vi "Get Antidoc Project Classes.vi"(8 "error in (no error)":errorcluster) -> (0 "error out":errorcluster, 2 "Config":refnum<class "Config.lvclass">, 3 "Document Type out":refnum<class "Document Type.lvclass">)   [LabVIEW 2020, in "CICD.lvlib"]
uses:
  CICD.lvlib
  <vilib>/Wovalab/AntiDoc/Document Type/Document/Document Type.lvclass
  <vilib>/Wovalab/AntiDoc/Document Type/Config/Config.lvclass
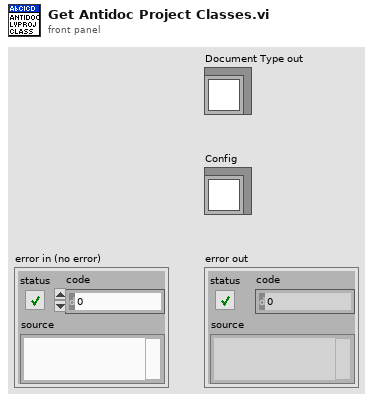
[diagram p1: front panel]
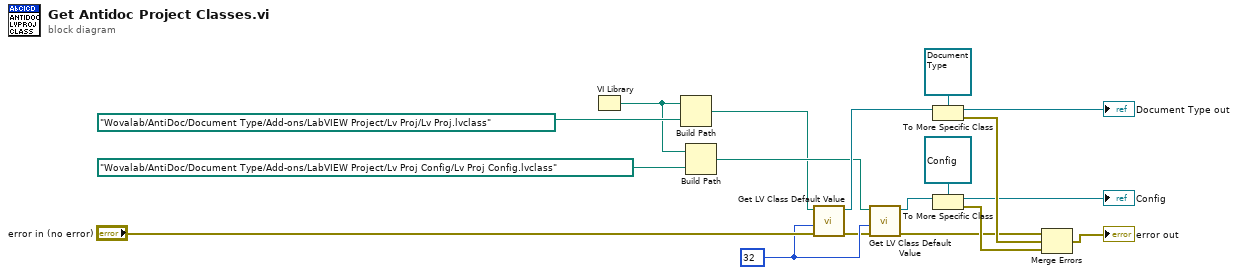
[diagram p0: block diagram]
diagram:
  w5 = u32 32 ("options")
  n1 = VI Library() -> (path=w1:path)
  n2 = Build Path(base path=w1, name or relative path=path "Wovalab/AntiDoc/Document Type/Add-ons/LabVIEW Project/Lv Proj/Lv Proj.lvclass") -> (appended path=w7:path)
  n3 = Build Path(base path=w1, name or relative path=path "Wovalab/AntiDoc/Document Type/Add-ons/LabVIEW Project/Lv Proj Config/Lv Proj Config.lvclass") -> (appended path=w8:path)
  n4 = call <vilib>:"Get LV Class Default Value.vi"("error in (no error)"="error in (no error)", "options"=w5, "class path"=w7) -> ("error out"=w4:errorcluster, "object"=w13:refnum<class>)  [unwired: 7 in]
  n5 = call <vilib>:"Get LV Class Default Value.vi"("error in (no error)"=w4, "options"=w5, "class path"=w8) -> ("error out"=w15:errorcluster, "object"=w14:refnum<class>)  [unwired: 7 in]
  n6 = To More Specific Class(target class=refnum<class "Document Type.lvclass"> refnum ("Document Type"), reference=w13) -> (specific class reference=→"Document Type out":refnum<class "Document Type.lvclass">, error out=w16:errorcluster)  [unwired: 1 in]
  n7 = To More Specific Class(target class=refnum<class "Config.lvclass"> refnum ("Config"), reference=w14) -> (specific class reference=→"Config":refnum<class "Config.lvclass">, error out=w17:errorcluster)  [unwired: 1 in]
  n8 = Merge Errors(w15, w16, w17) -> (→"error out":errorcluster)
